vi "Read JSON Tree.vi"(8 "error in (no error)":errorcluster, 11 "params in":refnum<class "params.lvclass">) -> (0 "error out":errorcluster, 2 "JSON Tree":variant, 3 "params out":refnum<class "params.lvclass">)   [LabVIEW 2015]
uses:
  params.lvclass
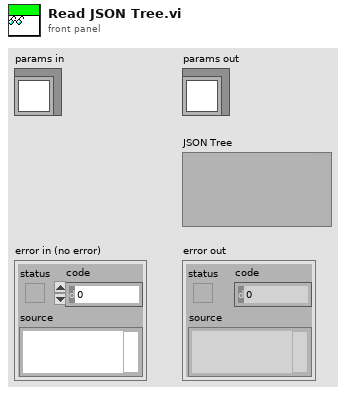
[diagram p1: front panel]
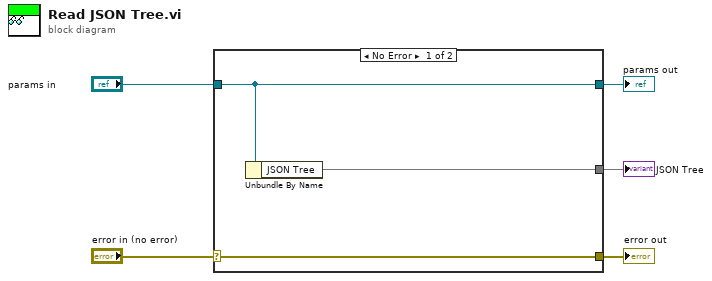
[diagram p0: block diagram]
diagram:
  n1 = case shown="No Error" "error in (no error)" {
    selector: "error in (no error)" -> [w8 w9]
    tunnel: [w8 w9] -> w4
    tunnel: [w7 w10] -> w2
    tunnel: "params in" -> [w7 w10]
    tunnel: [w6 _] -> w1
    frame No Error {
      n2 = Unbundle By Name(w7) -> ("JSON Tree"=w6)
    }
    frame Error {
    }
  }
  "error out" <- w4
  "params out" <- w2
  "JSON Tree" <- w1
